vi "Pack for gRPC.vi"(8 "error in":errorcluster, 9 "configuration / results":enum16{"Configuration", "Results"}(ring), 10 "data value":variant, 11 "measurement customizations in":refnum<class "Measurement Plugin.lvclass">) -> (0 "error out":errorcluster, 2 "any":T1, 3 "measurement customizations out":refnum<class "Measurement Plugin.lvclass">)   [LabVIEW 2021, in "Sweep_Channel Ganging.lvlib" / "Measurement Plugin.lvclass"]
uses:
  Measurement Plugin.lvclass
  Measurement Plugin.lvclass/Measurement Plugin.ctl
  Measurement Configuration.ctl
  Sweep_Channel Ganging.lvlib
  Measurement Results.ctl
  a6012965-5700-4384-8228-972e71b6560c.vi
  2eca732d-dbaa-43bf-a7dd-ede2da65bc1b.vi
  <vilib>/Plug-In SDKs/Measurements/Measurement Plugin Service/Measurement Plugin Service.lvclass
  C:/Program Files/National Instruments/LabVIEW 2021/vi.lib/Plug-In SDKs/Measurements/Measurement Plugin Service/Measurement Plugin Service.lvclass
  C:/Users/ngoli/Documents/pmic-labview/source/channel ganging/sweep channel ganging/Sweep_Channel Ganging/Advanced/Measurement Plugin.lvclass
  <vilib>/gRPC/LabVIEW gRPC Library/Shared/Any.ctl
  <vilib>/gRPC/LabVIEW gRPC Library/grpc-lvsupport-release.lvlib
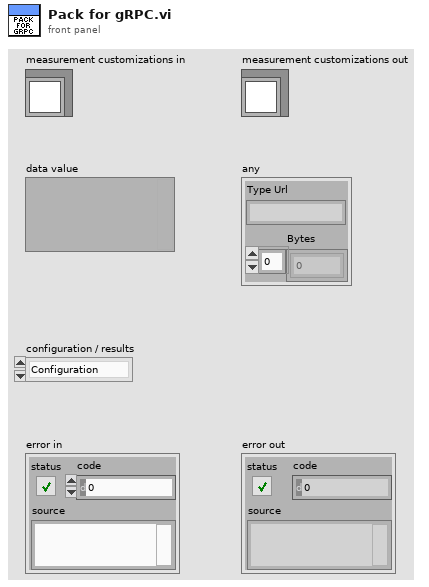
[diagram p1: front panel]
types:
  T1 = typedef "grpc-lvsupport-release.lvlib/Any.ctl" = cluster{"Type Url":string, "Bytes":u8[]}
  T2 = typedef "grpc-lvsupport-release.lvlib/grpcId.ctl" = u64
  T3 = typedef "Sweep_Channel Ganging.lvlib/Measurement Configuration.ctl" = cluster{"Source enable/disable":bool, "Load enable/disable":bool, "Source master resource name":string, "Source slave resource names":string[], "Load master resource name":string, "Load slave resource names":string[], "Source system configuration":enum32{"Series", "Parallel", "Manual"}, "Source output functio n":i32, "Source sweep scale":string, "Source start level":dbl, "Source stop level":dbl, "Source sweep points/points per decade":i32, "Source voltage/current level range":dbl, "Source sense":i32, "Source limit symmetry":enum32{"Symmetric", "Asymmetric"}, "Source current/voltage limit range":dbl, "Source current/voltage limit low":dbl, "Source current/voltage limit high":dbl, "Source source delay":dbl, "Source aperture time":dbl, "Source transient response":i32, "Source voltage gain bandwidth":dbl, "Source voltage compensation frequency":dbl, "Source voltage pole-zero ratio":dbl, "Source current gain bandwidth":dbl, "Source current compensation frequency":dbl, "Source current pole-zero ratio":dbl, "Load system configuration":enum32{"Series", "Parallel", "Manual"}, "Load output function":i32, "Load sweep scale":string, "Load start level":dbl, "Load stop level":dbl, "Load sweep points/points per decade":i32, "Load voltage/current level range":dbl, "Load sense":i32, "Load limit symmetry":enum32{"Symmetric", "Asymmetric"}, "Load current/voltage limit range":dbl, "Load current/voltage limit low":dbl, "Load current/voltage limit high":dbl, "Load source delay":dbl, "Load aperture time":dbl, "Load transient response":i32, "Load voltage gain bandwidth":dbl, "Load voltage compensation frequency":dbl, "Load voltage pole-zero ratio":dbl, "Load current gain bandwidth":dbl, "Load current compensation frequency":dbl, "Load current pole-zero ratio":dbl, "Load source trigger":string, "Load measure trigger":string}
  T4 = typedef "Sweep_Channel Ganging.lvlib/Measurement Results.ctl" = cluster{"Source sweep points":i32, "Load sweep points":i32, "Source sweep values":dbl[], "Ganged source voltages":dbl[], "Ganged source currents":dbl[], "Ganged load voltages":dbl[], "Ganged load currents":dbl[]}
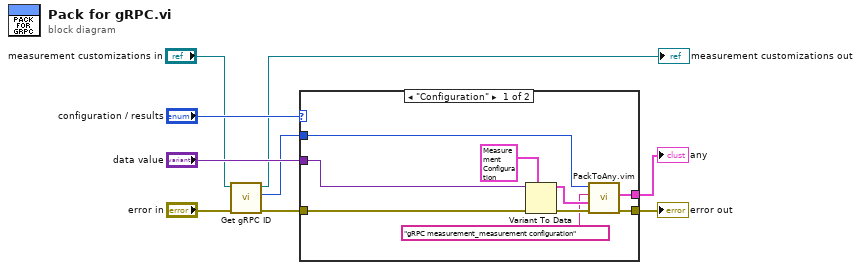
[diagram p0: block diagram]
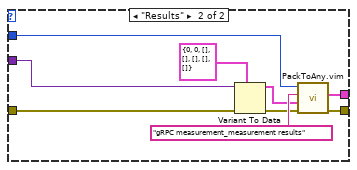
[diagram p2: hidden frame]
diagram:
  n1 = call <vilib>:"Get gRPC ID.vi"("error in"="error in", "measurement plugin service in"="measurement customizations in") -> ("error out"=w4:errorcluster, "gRPC ID"=w1:T2, "measurement plugin service out"=→"measurement customizations out":refnum<class "Measurement Plugin.lvclass">)  [unwired: 7 in]
  n2 = case shown="\"Configuration\"" "configuration / results" {
    tunnel: w4 -> [w18 w27]
    tunnel: "data value" -> [w17 w26]
    tunnel: w1 -> [w14 w22]
    tunnel: [w16 w24] -> w8
    tunnel: [w15 w23] -> w7
    frame "Configuration" {
      n3 = Variant To Data(error in=w18, type=T3 {"Source enable/disable"=FALSE, "Load enable/disable"=FALSE, "Source master resource name"="", "Source slave resource names"=[], "Load master resource name"="", "Load slave resource names"=[], "Source system configuration"=enum."Parallel", "Source output functio n"=1, "Source sweep scale"="Logarithmic", "Source start level"=0.005, "Source stop level"=6.0, "Source sweep points/points per decade"=14, "Source voltage/current level range"=4.0, "Source sense"=1009, "Source limit symmetry"=enum."Asymmetric", "Source current/voltage limit range"=20.0, "Source current/voltage limit low"=25.0, "Source current/voltage limit high"=-0.6, "Source source delay"=25.0, "Source aperture time"=1.0, "Source transient response"=1038, "Source voltage gain bandwidth"=2000.0, "Source voltage compensation frequency"=3530.0, "Source voltage pole-zero ratio"=2.0, "Source current gain bandwidth"=20000.0, "Source current compensation frequency"=4000.0, "Source current pole-zero ratio"=1.0, "Load system configuration"=enum."Parallel", "Load output function"=50, "Load sweep scale"="Logarithmic", "Load start level"=0.005, "Load stop level"=80.0, "Load sweep points/points per decade"=6, "Load voltage/current level range"=0.0, "Load sense"=1009, "Load limit symmetry"=enum."Symmetric", "Load current/voltage limit range"=inf, "Load current/voltage limit low"=10.0, "Load current/voltage limit high"=inf, "Load source delay"=0.005, "Load aperture time"=0.005, "Load transient response"=1038, "Load voltage gain bandwidth"=10000.0, "Load voltage compensation frequency"=50000.0, "Load voltage pole-zero ratio"=12.0, "Load current gain bandwidth"=14000.0, "Load current compensation frequency"=180000.0, "Load current pole-zero ratio"=0.3, "Load source trigger"="", "Load measure trigger"=""} ("measurement configuration"), Variant=w17) -> (data=w13:T3, error out=w12:errorcluster)
      n4 = call "PackToAny.vim"("error in"=w12, "Data To Pack"=w13, "Message Type"="gRPC measurement_measurement configuration", "gRPCid in"=w14) -> ("error out"=w16:errorcluster, "Any"=w15:T1)  [unwired: 5 in, 1 out]
    }
    frame "Results" {
      n5 = Variant To Data(error in=w27, type=T4 {"Source sweep points"=0, "Load sweep points"=0, "Source sweep values"=[], "Ganged source voltages"=[], "Ganged source currents"=[], "Ganged load voltages"=[], "Ganged load currents"=[]} ("Measurement Results"), Variant=w26) -> (data=w20:T4, error out=w19:errorcluster)
      n6 = call "PackToAny.vim"("error in"=w19, "Data To Pack"=w20, "Message Type"="gRPC measurement_measurement results", "gRPCid in"=w22) -> ("error out"=w24:errorcluster, "Any"=w23:T1)  [unwired: 5 in, 1 out]
    }
  }
  "error out" <- w8
  "any" <- w7
